vi "NI 9775 PD Demodulation (Host).vi"() -> ()   [LabVIEW 2021]
uses:
  <vilib>/userDefined/High Color/nirio_resource_hc.ctl
  <vilib>/LabVIEW Targets/FPGA/cRIO/shared/nicrio_ModuleControls/nicrio_cRIO-9775_ContinuousDataRates4ChansRing.ctl
  <vilib>/LabVIEW Targets/FPGA/cRIO/shared/nicrio_ModuleControls/nicrio_BasicConversionTime.ctl
  <vilib>/Utility/file.llb/Write Delimited Spreadsheet (DBL).vi
  <vilib>/FPGAPlugInAG/cRIO-9053/niLvFpga_Open_cRIO-9053.vi
  <vilib>/rvi/interface/common/dynamic/niFpgaDynamicAddResources.vi
  <vilib>/FPGAPlugInAG/Dynamic/niLvFpga_Reset_Dynamic.vi
  <vilib>/Utility/error.llb/Error Cluster From Error Code.vi
  <vilib>/rvi/errors/niLvFpgaAdjustHostInterfaceError.vi
  <vilib>/FPGAPlugInAG/Dynamic/niLvFpga_Run_Dynamic.vi
  <vilib>/FPGAPlugInAG/Dynamic/niLvFpga_Close_Dynamic.vi
  <vilib>/rvi/interface/nirviOpenFPGA/nirviOpenFPGA.xnode
  FPGA Bitfiles/ni9775crio9053_FPGATarget2_NI9775GettingSta_I+1qGd-Sz4M.lvbitx
  <vilib>/rvi/interface/nirviMethod/nirviMethod.xnode
  <vilib>/rvi/interface/nirviReadWriteControl/nirviReadWriteControl.xnode
  <vilib>/rvi/interface/nirviCloseFPGA/nirviCloseFPGA.xnode
  <vilib>/rvi/interface/Simulation/niFpgaSimulationCallBeginRW.vi
  <vilib>/FPGAPlugInAG/Dynamic/niLvFpga_ReadFifo_Dynamic.vi
  <vilib>/rvi/errors/niLvFpgaMergeErrorWithErrorCode.vi
  NiFpgaLv.dll
panel:
  in  "Save":bool
  in  "stop":bool
  in  "?":T1(tab)=enum."Demodulated"
  out "Raw Signal":waveform(dbl)[](graph)=[{"t0"=timestamp(0 s since 1904-01-01), "dt"=8e-05, "Y"=array[1241 elements]}, {"t0"=timestamp(0 s since 1904-01-01), "dt"=8e-05, "Y"=array[1241 elements]}, {"t0"=timestamp(0 s since 1904-01-01), "dt"=8e-05, "Y"=array[1241 elements]}, {"t0"=timestamp(0 s since 1904-01-01), "dt"=8e-05, "Y"=array[1241 elements]}]
  out "Num pts Pos":i32=3
  out "Num pts Neg":i32=3
  out "Low level":bool
  out "High level":bool=TRUE
  out "Num pts Neg 2":i32=3
  out "Num pts Pos 2":i32=3
  out "Num pts Neg 3":i32=3
  out "Num pts Pos 3":i32=3
  out "Num pts Pos 4":i32=3
  out "Num pts Neg 4":i32=3
  out "Demodulated signal 4":dbl(graph)
  out "Demodulated signal 3":dbl(graph)=0.400634765625
  out "Demodulated signal 1":dbl(graph)=0.0013427734375
  out "Demodulated signal 2":dbl(graph)=0.0006103515625
  out "Normalized signal 3":dbl(graph)
  out "Normalized signal 1":dbl(graph)
  out "Normalized signal 2":dbl(graph)
  out "?":cluster{dbl[], dbl[]}(graph)
  in  "Draw Lissajous":bool
  out "Modulation frequency":dbl=2083.3333333333335
  in  "Filename":path=path "C:/Users/data/2023_09_14_NI9230_pd-demodulation-12_8ks_100Hzmod_85mA_10c_ch1_demod1_ch2_demod2_ch3_demodpower_mid1_mid3_001.lvm"
  out "Arrays in queue":i32
  in  "Consumer loop update rate (ms)":u32=10
  out "Consumer loop time":u32=100
  out "Sample Rate":dbl=12500.0
  out "Producer loop time":u32=100
  in  "Enable Low Pass Filter":T2={"Enable Low Pass Filter CH1"=TRUE, "Enable Low Pass Filter CH2"=TRUE, "Enable Low Pass Filter CH3"=TRUE, "Enable Low Pass Filter CH0"=TRUE}
  in  "Timing Mode":T3=enum."High Resolution"
  in  "Continuous Data Rate":T4=1600 items=["1.000 MS/s (NI 9775)"=20, "833.333 KS/s (NI 9775)"=24, "714.286 KS/s (NI 9775)"=28, "625.000 KS/s (NI 9775)"=32, "555.556 KS/s (NI 9775)"=36, "500.000 KS/s (NI 9775)"=40, "454.545 KS/s (NI 9775)"=44, "416.667 KS/s (NI 9775)"=48, "384.615 KS/s (NI 9775)"=52, "357.143 KS/s (NI 9775)"=56, "333.333 KS/s (NI 9775)"=60, "312.500 KS/s (NI 9775)"=64, "294.118 KS/s (NI 9775)"=68, "277.778 KS/s (NI 9775)"=72, "263.158 KS/s (NI 9775)"=76, "250.000 KS/s (NI 9775)"=80, "238.095 KS/s (NI 9775)"=84, "227.273 KS/s (NI 9775)"=88, "217.391 KS/s (NI 9775)"=92, "208.333 KS/s (NI 9775)"=96, "200.000 KS/s (NI 9775)"=100, "192.308 KS/s (NI 9775)"=104, "185.185 KS/s (NI 9775)"=108, "178.571 KS/s (NI 9775)"=112, "172.414 KS/s (NI 9775)"=116, "166.667 KS/s (NI 9775)"=120, "161.290 KS/s (NI 9775)"=124, "156.250 KS/s (NI 9775)"=128, "151.515 KS/s (NI 9775)"=132, "147.059 KS/s (NI 9775)"=136, "142.857 KS/s (NI 9775)"=140, "138.889 KS/s (NI 9775)"=144, "135.135 KS/s (NI 9775)"=148, "131.579 KS/s (NI 9775)"=152, "128.205 KS/s (NI 9775)"=156, "125.000 KS/s (NI 9775)"=160, "121.951 KS/s (NI 9775)"=164, "119.048 KS/s (NI 9775)"=168, "116.279 KS/s (NI 9775)"=172, "113.636 KS/s (NI 9775)"=176, "111.111 KS/s (NI 9775)"=180, "108.696 KS/s (NI 9775)"=184, "106.383 KS/s (NI 9775)"=188, "104.167 KS/s (NI 9775)"=192, "102.041 KS/s (NI 9775)"=196, "100.000 KS/s (NI 9775)"=200, "50.000 KS/s (NI 9775)"=400, "33.333 KS/s (NI 9775)"=600, "25.000 KS/s (NI 9775)"=800, "20.000 KS/s (NI 9775)"=1000, "16.667 KS/s (NI 9775)"=1200, "14.286 KS/s (NI 9775)"=1400, "12.500 KS/s (NI 9775)"=1600, "11.111 KS/s (NI 9775)"=1800, "10.000 KS/s (NI 9775)"=2000, "9.091 KS/s (NI 9775)"=2200, "8.333 KS/s (NI 9775)"=2400, "7.692 KS/s (NI 9775)"=2600, "7.143 KS/s (NI 9775)"=2800, "6.667 KS/s (NI 9775)"=3000, "6.250 KS/s (NI 9775)"=3200, "5.882 KS/s (NI 9775)"=3400, "5.556 KS/s (NI 9775)"=3600, "5.000 KS/s (NI 9775)"=4000, "4.762 KS/s (NI 9775)"=4200, "4.545 KS/s (NI 9775)"=4400, "4.348 KS/s (NI 9775)"=4600, "4.167 KS/s (NI 9775)"=4800, "4.000 KS/s (NI 9775)"=5000, "3.846 KS/s (NI 9775)"=5200, "3.571 KS/s (NI 9775)"=5600, "3.333 KS/s (NI 9775)"=6000, "3.125 KS/s (NI 9775)"=6400, "2.941 KS/s (NI 9775)"=6800, "2.778 KS/s (NI 9775)"=7200, "2.632 KS/s (NI 9775)"=7600, "2.500 KS/s (NI 9775)"=8000, "2.381 KS/s (NI 9775)"=8400, "2.273 KS/s (NI 9775)"=8800, "2.174 KS/s (NI 9775)"=9200, "2.083 KS/s (NI 9775)"=9600, "2.000 KS/s (NI 9775)"=10000, "1.923 KS/s (NI 9775)"=10400, "1.852 KS/s (NI 9775)"=10800, "1.786 KS/s (NI 9775)"=11200, "1.724 KS/s (NI 9775)"=11600, "1.667 KS/s (NI 9775)"=12000, "1.613 KS/s (NI 9775)"=12400, "1.563 KS/s (NI 9775)"=12800, "1.515 KS/s (NI 9775)"=13200, "1.471 KS/s (NI 9775)"=13600, "1.429 KS/s (NI 9775)"=14000, "1.389 KS/s (NI 9775)"=14400, "1.351 KS/s (NI 9775)"=14800, "1.316 KS/s (NI 9775)"=15200, "1.282 KS/s (NI 9775)"=15600, "1.250 KS/s (NI 9775)"=16000, "1.220 KS/s (NI 9775)"=16400, "1.190 KS/s (NI 9775)"=16800, "1.163 KS/s (NI 9775)"=17200, "1.136 KS/s (NI 9775)"=17600, "1.111 KS/s (NI 9775)"=18000, "1.087 KS/s (NI 9775)"=18400, "1.064 KS/s (NI 9775)"=18800, "1.042 KS/s (NI 9775)"=19200, "1.020 KS/s (NI 9775)"=19600, "1.000 KS/s (NI 9775)"=20000, "0.980 KS/s (NI 9775)"=20400, "0.962 KS/s (NI 9775)"=20800, "0.943 KS/s (NI 9775)"=21200, "0.926 KS/s (NI 9775)"=21600, "0.909 KS/s (NI 9775)"=22000, "0.893 KS/s (NI 9775)"=22400, "0.877 KS/s (NI 9775)"=22800, "0.862 KS/s (NI 9775)"=23200, "0.847 KS/s (NI 9775)"=23600, "0.833 KS/s (NI 9775)"=24000, "0.820 KS/s (NI 9775)"=24400, "0.806 KS/s (NI 9775)"=24800, "0.794 KS/s (NI 9775)"=25200, "0.781 KS/s (NI 9775)"=25600, "0.694 KS/s (NI 9775)"=28800, "0.625 KS/s (NI 9775)"=32000, "0.568 KS/s (NI 9775)"=35200, "0.521 KS/s (NI 9775)"=38400, "0.446 KS/s (NI 9775)"=44800, "0.391 KS/s (NI 9775)"=51200, "0.347 KS/s (NI 9775)"=57600, "0.313 KS/s (NI 9775)"=64000]
  out "Host error out":errorcluster
  out "FPGA error out":errorcluster
  out "FIFO":u32=4
  out "Data FIFO Full":bool
  in  "Read FIFO update rate (ms)":u32=100
  in  "RIO Device":T5="RIO0"
  # "FPGA Input Parameters"
  # "Timing Parameters"
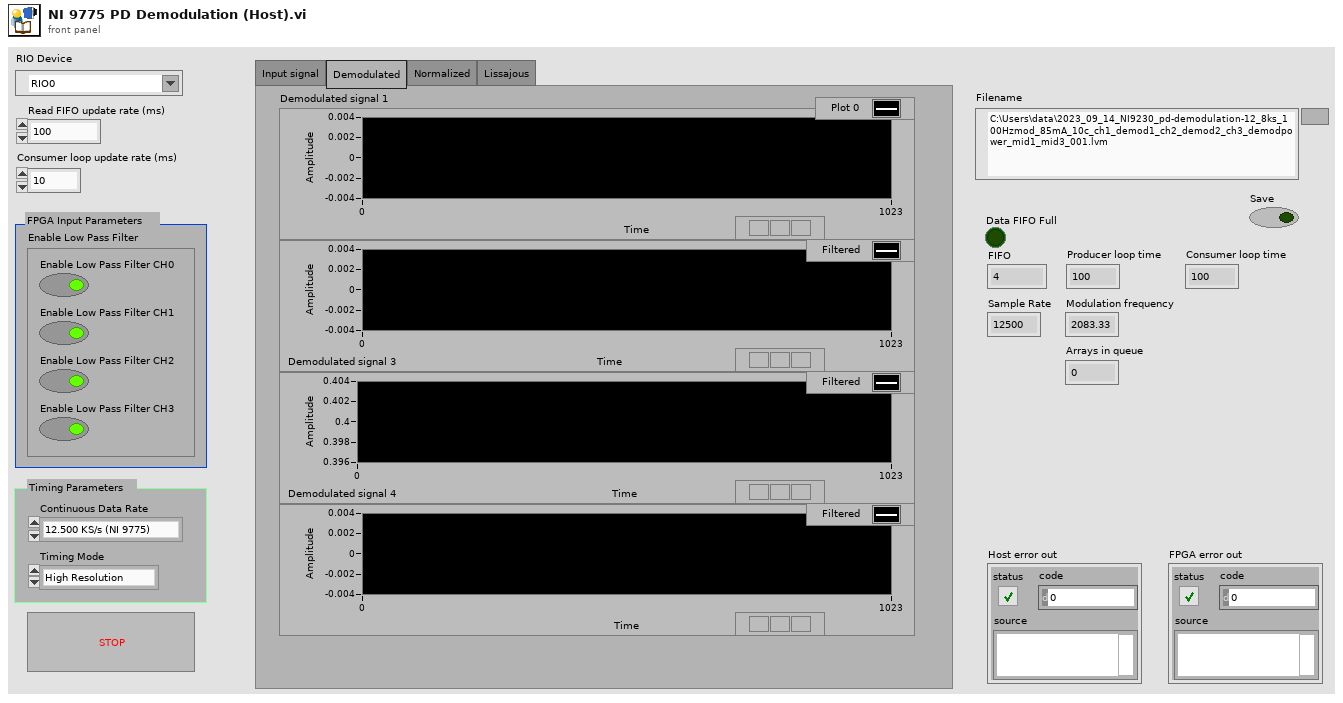
[diagram p1: front panel]
types:
  T1 = enum32{"Input signal", "Demodulated", "Normalized", "Lissajous"}
  T2 = cluster{"Enable Low Pass Filter CH1":bool, "Enable Low Pass Filter CH2":bool, "Enable Low Pass Filter CH3":bool, "Enable Low Pass Filter CH0":bool}
  T3 = typedef "nicrio_BasicConversionTime.ctl" = enum8{"High Speed", "High Resolution"}
  T4 = typedef "nicrio_cRIO-9775_ContinuousDataRates4ChansRing.ctl" = u16
  T5 = typedef "nirio_resource_hc.ctl" = tag
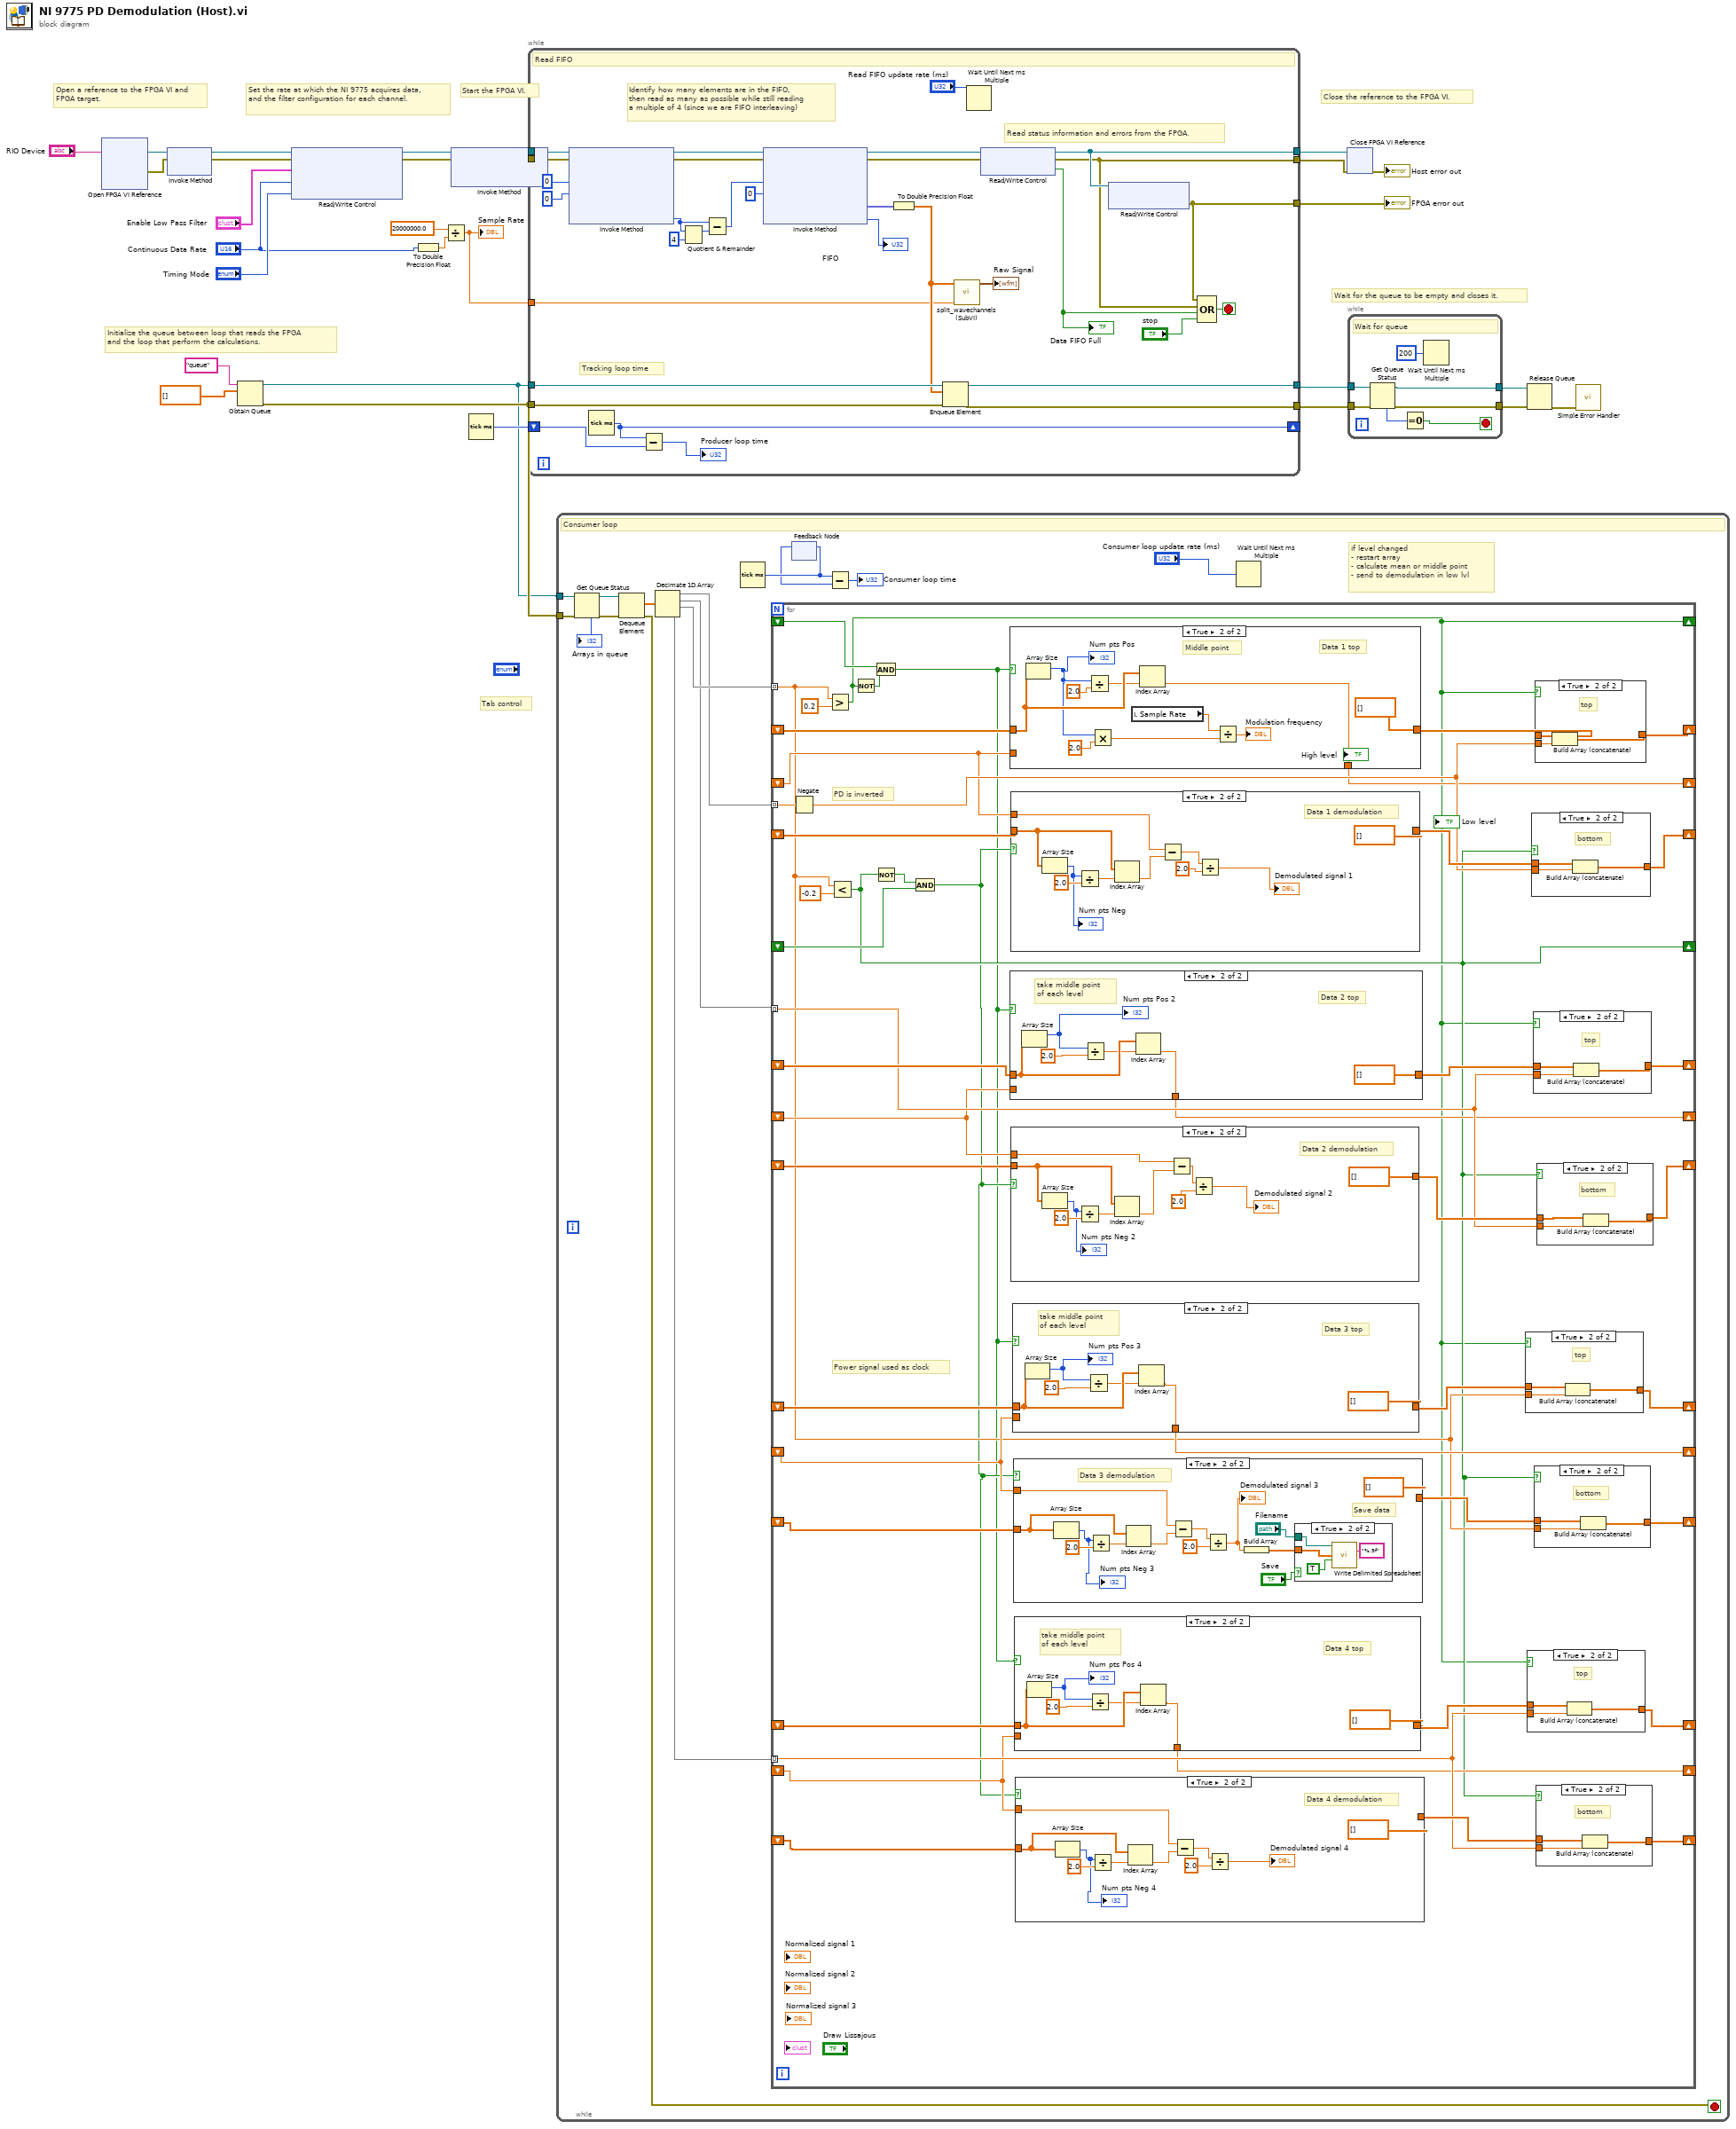
[diagram p0: block diagram]
diagram:
  # "Tab control"
  # "Initialize the queue between loop that reads the FPGA\nand the loop that perform the calculations."
  # "Wait for the queue to be empty and closes it."
  # "Close the reference to the FPGA VI."
  # "Start the FPGA VI."
  # "Set the rate at which the NI 9775 acquires data, and the filter configuration for each channel."
  # "Open a reference to the FPGA VI and FPGA target."
  n1 = xnode "Open FPGA VI Reference"("resource name"="RIO Device") -> ("FPGA VI Reference Out"=w17:refnum<k20>, "error out"=w16:errorcluster)  [unwired: 1 in]
  n2 = xnode "Invoke Method"("FPGA VI Reference In"=w17, "error in"=w16) -> ("FPGA VI Reference Out"=w21:refnum<k20>, "error out"=w22:errorcluster)
  n3 = Obtain Queue(name (unnamed)="queue", element data type=dbl[] []) -> (queue out=w1:refnum<queue>, error out=w2:errorcluster)  [unwired: 3 in, 1 out]
  n4 = xnode "Read/Write Control"("FPGA VI Reference In"=w21, "error in"=w22, "Enable Low Pass Filter"="Enable Low Pass Filter", "Continuous Data Rate"="Continuous Data Rate", "Timing Mode"="Timing Mode") -> ("FPGA VI Reference Out"=w25:refnum<k20>, "error out"=w26:errorcluster)
  n5 = To Double Precision Float(number="Continuous Data Rate") -> (double precision float=w5:dbl)
  n6 = Divide(x=20000000.0, y=w5) -> (x/y=w3:dbl)
  "Sample Rate" <- w3
  n7 = xnode "Invoke Method"("FPGA VI Reference In"=w25, "error in"=w26) -> ("FPGA VI Reference Out"=w28:refnum<k20>, "error out"=w29:errorcluster)  [unwired: 1 in]
  n8 = Tick Count (ms)() -> (millisecond timer value=w7:u32)
  n9 = while {
    tunnel: w29 -> [w44]
    tunnel: w28 -> [w45]
    tunnel: [w53] -> w27
    tunnel: [w52] -> w24
    tunnel: [w51] -> w20
    tunnel: w1 -> [w39]
    tunnel: [w38] -> w12
    tunnel: w2 -> [w37]
    tunnel: [w36] -> w10
    shift-right: [w34] -> _
    shift-left: w7 -> [w33]
    tunnel: w3 -> [w31]
    stop <- w61 stop-if-true
    # "Tracking loop time"
    # "Read status information and errors from the FPGA."
    # "Identify how many elements are in the FIFO, \nthen read as many as possible while still reading\na multiple of 4 (since we are FIFO interleaving)"
    # "Read FIFO"
    n10 = xnode "Invoke Method"("FPGA VI Reference In"=w45, "error in"=w44, "Number of Elements"=u32 0, "Timeout (ms)"=0) -> ("FPGA VI Reference Out"=w43:refnum<k20>, "error out"=w42:errorcluster, "Elements Remaining"=w46:u32)  [unwired: 1 out]
    n11 = Tick Count (ms)() -> (millisecond timer value=w34:u32)
    n12 = Subtract(x=w34, y=w33) -> (x-y=→"Producer loop time":u32)
    n13 = Quotient & Remainder(x=w46, y=u32 4) -> (x-y*floor(x/y)=w47:u32)  [unwired: 1 out]
    n14 = Subtract(x=w46, y=w47) -> (x-y=w41:u32)
    n15 = xnode "Invoke Method"("FPGA VI Reference In"=w43, "error in"=w42, "Number of Elements"=w41, "Timeout (ms)"=0 ("Timeout")) -> ("FPGA VI Reference Out"=w58:refnum<k20>, "error out"=w57:errorcluster, "Data"=w54:fxp<+/-,17,5>[], "Elements Remaining"=→"FIFO":u32)
    n16 = To Double Precision Float(number=w54) -> (double precision float=w32:dbl[])
    n17 = Enqueue Element(queue=w39, element=w32, error in (no error)=w37) -> (queue out=w38:refnum<queue>, error out=w36:errorcluster)  [unwired: 1 in, 1 out]
    n18 = call "split_wavechannels (SubVI).vi"("Sample rate"=w31, "Array in"=w32) -> ("Array out"=→"Raw Signal":waveform(dbl)[])  [unwired: 9 in]
    n19 = Wait Until Next ms Multiple(millisecond multiple="Read FIFO update rate (ms)") -> ()  [unwired: 1 out]
    n20 = xnode "Read/Write Control"("FPGA VI Reference In"=w58, "error in"=w57) -> ("FPGA VI Reference Out"=w53:refnum<k20>, "error out"=w52:errorcluster, "Data FIFO Full"=w60:bool)
    "Data FIFO Full" <- w60
    n21 = xnode "Read/Write Control"("FPGA VI Reference In"=w53) -> ("FPGA Error Out"=w51:errorcluster)  [unwired: 1 in, 2 out]
    n22 = Compound Arithmetic op=OR(w51, w52, w60, "stop") -> (w61:bool)
  }
  "FPGA error out" <- w20
  n23 = while {
    tunnel: w1 -> [w72]
    tunnel: w2 -> [w73]
    stop <- w74 stop-if-true
    # "if level changed\n- restart array\n- calculate mean or middle point\n- send to demodulation in low lvl"
    # "Consumer loop"
    n24 = Get Queue Status(queue=w72, error in (no error)=w73) -> (queue out=w71:refnum<queue>, error out=w70:errorcluster, # elements in queue=→"Arrays in queue":i32)  [unwired: 1 in, 5 out]
    n25 = Dequeue Element(queue=w71, error in (no error)=w70) -> (element=w69:dbl[], error out=w74:errorcluster)  [unwired: 1 in, 2 out]
    n26 = Decimate 1D Array(w69) -> (w65:dbl[], w66:dbl[], w67:dbl[], w62:dbl[])
    n27 = Tick Count (ms)() -> (millisecond timer value=w64:u32)
    n28 = for {
      tunnel: w67 -> [w90] mode=indexing
      shift-right: [w79] -> _
      shift-left: _ -> [w120]
      shift-right: [w80] -> _
      shift-left: _ -> [w98]
      shift-right: [w117] -> _
      shift-left: _ -> [w119]
      shift-right: [w118] -> _
      shift-left: _ -> [w114]
      tunnel: w65 -> [w101] mode=indexing
      tunnel: w66 -> [w95] mode=indexing
      shift-right: [w111] -> _
      shift-left: _ -> [w112]
      shift-right: [w110] -> _
      shift-left: _ -> [w108]
      shift-right: [w105] -> _
      shift-left: _ -> [w106]
      shift-right: [w103] -> _
      shift-left: _ -> [w102]
      shift-right: [w97] -> _
      shift-left: _ -> [w96]
      shift-right: [w94] -> _
      shift-left: _ -> [w91]
      shift-right: [w93] -> _
      shift-left: _ -> [w92]
      tunnel: w62 -> [w87] mode=indexing
      shift-right: [w82] -> _
      shift-left: _ -> [w86]
      shift-right: [w85] -> _
      shift-left: _ -> [w81]
      shift-right: [w84] -> _
      shift-left: _ -> [w83]
      # "PD is inverted"
      # "Power signal used as clock"
      n29 = Negate(x=w101) -> (-x=w100:dbl)
      n30 = Greater?(x=w90, y=0.2) -> (0:w79:bool)
      n31 = Less?(x=w90, y=-0.2) -> (x < y?=w80:bool)
      n32 = Not(x=w79) -> (.not. x?=w122:bool)
      n33 = And(x=w120, y=w122) -> (x .and. y?=w77:bool)
      n34 = Not(x=w80) -> (.not. x?=w99:bool)
      n35 = And(x=w99, y=w98) -> (x .and. y?=w78:bool)
      n36 = case shown="True" w77 {
        tunnel: [w171 dbl[] []] -> w115
        tunnel: w114 -> [w171 w178]
        tunnel: [w170 w175] -> w97
        tunnel: w96 -> [w170 _]
        frame False {
        }
        frame True {
          # "Middle point"
          # "Data 1 top"
          n37 = Array Size(array=w178) -> (size(s)=w172:i32)
          "Num pts Pos" <- w172
          n38 = Divide(x=w172, y=2.0) -> (x/y=w177:dbl)
          n39 = Multiply(x=w172, y=2.0) -> (x*y=w179:dbl)
          n40 = local read "Sample Rate"() -> (w180:dbl)
          n41 = Index Array(array=w178, index=w177) -> (element=w175:dbl)
          n42 = Divide(x=w180, y=w179) -> (x/y=→"Modulation frequency":dbl)
        }
      }
      n43 = case shown="True" w77 {
        tunnel: [w152 dbl[] []] -> w113
        tunnel: w108 -> [w152 w156]
        tunnel: [w151 w154] -> w94
        tunnel: w91 -> [w151 _]
        frame False {
        }
        frame True {
          # "Data 2 top"
          # "take middle point \nof each level"
          n44 = Array Size(array=w156) -> (size(s)=w153:i32)
          "Num pts Pos 2" <- w153
          n45 = Divide(x=w153, y=2.0) -> (x/y=w155:dbl)
          n46 = Index Array(array=w156, index=w155) -> (element=w154:dbl)
        }
      }
      n47 = case shown="True" w78 {
        tunnel: [w182 dbl[] []] -> w116
        tunnel: w119 -> [w182 w186]
        tunnel: w96 -> [_ w185]
        frame False {
        }
        frame True {
          # "Data 1 demodulation"
          n48 = Array Size(array=w186) -> (size(s)=w183:i32)
          "Num pts Neg" <- w183
          n49 = Divide(x=w183, y=2.0) -> (x/y=w187:dbl)
          n50 = Index Array(array=w186, index=w187) -> (element=w189:dbl)
          n51 = Subtract(x=w185, y=w189) -> (x-y=w191:dbl)
          n52 = Divide(x=w191, y=2.0) -> (x/y=→"Demodulated signal 1":dbl)
        }
      }
      n53 = case shown="True" w78 {
        tunnel: [w159 dbl[] []] -> w109
        tunnel: w112 -> [w159 w163]
        tunnel: w91 -> [_ w162]
        frame False {
        }
        frame True {
          # "Data 2 demodulation"
          n54 = Array Size(array=w163) -> (size(s)=w160:i32)
          "Num pts Neg 2" <- w160
          n55 = Divide(x=w160, y=2.0) -> (x/y=w164:dbl)
          n56 = Index Array(array=w163, index=w164) -> (element=w166:dbl)
          n57 = Subtract(x=w162, y=w166) -> (x-y=w168:dbl)
          n58 = Divide(x=w168, y=2.0) -> (x/y=→"Demodulated signal 2":dbl)
        }
      }
      n59 = case shown="True" w77 {
        tunnel: [w194 dbl[] []] -> w107
        tunnel: w106 -> [w194 w198]
        tunnel: [w193 w196] -> w93
        tunnel: w92 -> [w193 _]
        frame False {
        }
        frame True {
          # "Data 3 top"
          # "take middle point \nof each level"
          n60 = Array Size(array=w198) -> (size(s)=w195:i32)
          "Num pts Pos 3" <- w195
          n61 = Divide(x=w195, y=2.0) -> (x/y=w197:dbl)
          n62 = Index Array(array=w198, index=w197) -> (element=w196:dbl)
        }
      }
      n63 = case shown="True" w78 {
        tunnel: [w201 dbl[] []] -> w104
        tunnel: w102 -> [w201 w208]
        tunnel: w92 -> [_ w207]
        frame False {
        }
        frame True {
          # "Save data"
          # "Data 3 demodulation"
          n64 = Array Size(array=w208) -> (size(s)=w206:i32)
          "Num pts Neg 3" <- w206
          n65 = Divide(x=w206, y=2.0) -> (x/y=w209:dbl)
          n66 = Index Array(array=w208, index=w209) -> (element=w211:dbl)
          n67 = Subtract(x=w207, y=w211) -> (x-y=w213:dbl)
          n68 = Divide(x=w213, y=2.0) -> (x/y=w203:dbl)
          "Demodulated signal 3" <- w203
          n69 = Build Array(w203) -> (w202:dbl[])
          n70 = case shown="True" "Save" {
            tunnel: "Filename" -> [_ w216]
            tunnel: w202 -> [_ w215]
            frame False {
            }
            frame True {
              n71 = call-poly <vilib>:"Write Delimited Spreadsheet.vi"("file path (dialog if empty)"=w216, "format (%.3f)"="%.9f", "1D data"=w215, "append to file? (new file:F)"=TRUE) -> ()  [unwired: 10 in, 2 out]
            }
          }
        }
      }
      n72 = case shown="True" w77 {
        tunnel: [w125 dbl[] []] -> w88
        tunnel: w86 -> [w125 w129]
        tunnel: [w124 w127] -> w84
        tunnel: w83 -> [w124 _]
        frame False {
        }
        frame True {
          # "Data 4 top"
          # "take middle point \nof each level"
          n73 = Array Size(array=w129) -> (size(s)=w126:i32)
          "Num pts Pos 4" <- w126
          n74 = Divide(x=w126, y=2.0) -> (x/y=w128:dbl)
          n75 = Index Array(array=w129, index=w128) -> (element=w127:dbl)
        }
      }
      n76 = case shown="True" w78 {
        tunnel: [w132 dbl[] []] -> w89
        tunnel: w81 -> [w132 w136]
        tunnel: w83 -> [_ w135]
        frame False {
        }
        frame True {
          # "Data 4 demodulation"
          n77 = Array Size(array=w136) -> (size(s)=w134:i32)
          "Num pts Neg 4" <- w134
          n78 = Divide(x=w134, y=2.0) -> (x/y=w137:dbl)
          n79 = Index Array(array=w136, index=w137) -> (element=w139:dbl)
          n80 = Subtract(x=w135, y=w139) -> (x-y=w141:dbl)
          n81 = Divide(x=w141, y=2.0) -> (x/y=→"Demodulated signal 4":dbl)
        }
      }
      n82 = case shown="True" w79 {
        tunnel: w107 -> [w239 w242]
        tunnel: [w239 w240] -> w105
        tunnel: w90 -> [_ w241]
        frame False {
        }
        frame True {
          # "top"
          n83 = Build Array (concatenate)(w242, w241) -> (w240:dbl[])
        }
      }
      n84 = case shown="True" w79 {
        tunnel: w88 -> [w147 w150]
        tunnel: [w147 w148] -> w82
        tunnel: w87 -> [_ w149]
        frame False {
        }
        frame True {
          # "top"
          n85 = Build Array (concatenate)(w150, w149) -> (w148:dbl[])
        }
      }
      n86 = case shown="True" w80 {
        tunnel: w116 -> [w227 w230]
        tunnel: w100 -> [_ w229]
        tunnel: [w227 w228] -> w117
        frame False {
        }
        frame True {
          # "bottom"
          n87 = Build Array (concatenate)(w230, w229) -> (w228:dbl[])
        }
      }
      n88 = case shown="True" w79 {
        tunnel: w113 -> [w223 w226]
        tunnel: [w223 w224] -> w110
        tunnel: w95 -> [_ w225]
        frame False {
        }
        frame True {
          # "top"
          n89 = Build Array (concatenate)(w226, w225) -> (w224:dbl[])
        }
      }
      n90 = case shown="True" w80 {
        tunnel: w104 -> [w235 w238]
        tunnel: [w235 w236] -> w103
        tunnel: w90 -> [_ w237]
        frame False {
        }
        frame True {
          # "bottom"
          n91 = Build Array (concatenate)(w238, w237) -> (w236:dbl[])
        }
      }
      n92 = case shown="True" w79 {
        tunnel: w115 -> [w231 w234]
        tunnel: [w231 w232] -> w118
        tunnel: w100 -> [_ w233]
        frame False {
        }
        frame True {
          # "top"
          n93 = Build Array (concatenate)(w234, w233) -> (w232:dbl[])
        }
      }
      n94 = case shown="True" w80 {
        tunnel: w89 -> [w143 w146]
        tunnel: [w143 w144] -> w85
        tunnel: w87 -> [_ w145]
        frame False {
        }
        frame True {
          # "bottom"
          n95 = Build Array (concatenate)(w146, w145) -> (w144:dbl[])
        }
      }
      n96 = case shown="True" w80 {
        tunnel: w109 -> [w219 w222]
        tunnel: [w219 w220] -> w111
        tunnel: w95 -> [_ w221]
        frame False {
        }
        frame True {
          # "bottom"
          n97 = Build Array (concatenate)(w222, w221) -> (w220:dbl[])
        }
      }
    }
    n98 = feedback #1() -> (w63:u32)  [unwired: 1 in]
    n99 = feedback-in #1(w64) -> ()
    n100 = Subtract(x=w64, y=w63) -> (x-y=→"Consumer loop time":u32)
    n101 = Wait Until Next ms Multiple(millisecond multiple="Consumer loop update rate (ms)") -> ()  [unwired: 1 out]
  }
  n102 = xnode "Close FPGA VI Reference"("FPGA VI Reference In"=w27, "error in"=w24) -> ("error out"=→"Host error out":errorcluster)
  n103 = while {
    tunnel: w12 -> [w249]
    tunnel: [w245] -> w11
    tunnel: w10 -> [w244]
    tunnel: [w243] -> w9
    stop <- w247 stop-if-true
    # "Wait for queue"
    n104 = Get Queue Status(queue=w249, error in (no error)=w244) -> (queue out=w245:refnum<queue>, error out=w243:errorcluster, # elements in queue=w248:i32)  [unwired: 1 in, 5 out]
    n105 = Equal To 0?(x=w248) -> (x = 0?=w247:bool)
    n106 = Wait Until Next ms Multiple(millisecond multiple=u32 200) -> ()  [unwired: 1 out]
  }
  n107 = Release Queue(queue=w11, error in (no error)=w9) -> (error out=w8:errorcluster)  [unwired: 1 in, 2 out]
  n108 = call <vilib>:"Simple Error Handler.vi"("error in (no error)"=w8) -> ()  [unwired: 4 in, 5 out]
